vi "textParsePowerBoard.vi"(8 "error in (no error)":errorcluster, 10 "file name":string, 11 "base path":path=path "C:/specsheetsController/Sheets/PowerBoard") -> (0 "error out":errorcluster, 2 "all rows":string[][](array[string]), 3 "appended path":path)   [LabVIEW 2018]
uses:
  <vilib>/Utility/file.llb/Read Delimited Spreadsheet (string).vi
  MotorController/#include/Global textParse.vi
panel:
  out "protocolGrade":string
  out "protocolDistance":string
  out "protocolResistance":string
  out "Sense Voltage Tol. Max":string
  out "Sense Voltage Tol. Min":string
  out "Sense Voltage":string
  out "Allowable Power Interuption":string
  out "Voltage Micro Tol. Max":string
  out "Voltage Micro Tol. Min":string
  out "Voltage Micro":string
  out "Rated Output Current Tol. Max":string
  out "Rated Output Current Tol. Min":string
  out "Rated Output Current":string
  out "Ripple/Noise Tol. Max":string
  out "Ripple/Noise Tol. Min":string
  out "Ripple/Noise":string
  out "Voltage Output Tol. Max":string
  out "Voltage  Output Tol. Min":string
  out "Voltage Output":string
  out "Max Input Current":string
  out "Input Current":string
  out "Input Voltage Tol. Max":string
  out "Input Voltage Tol. Min":string
  out "Input Voltage":string
  out "Firmware":string
  out "Part Number":string
  out "Part Name":string
  # "Global variables"
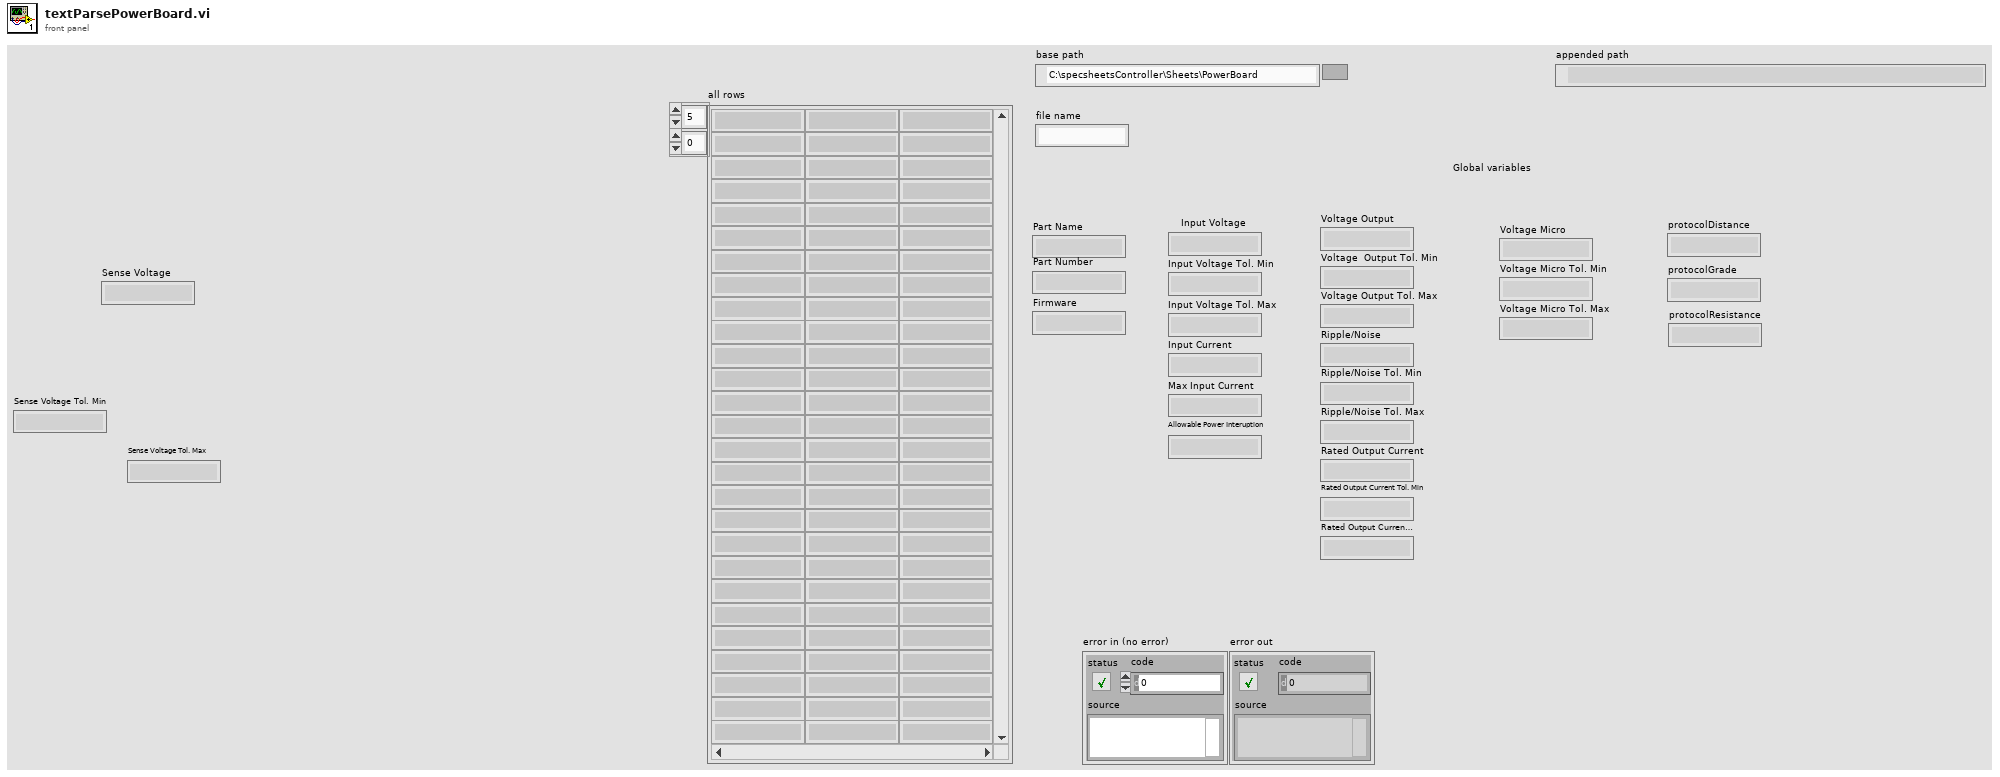
[diagram p1: front panel]
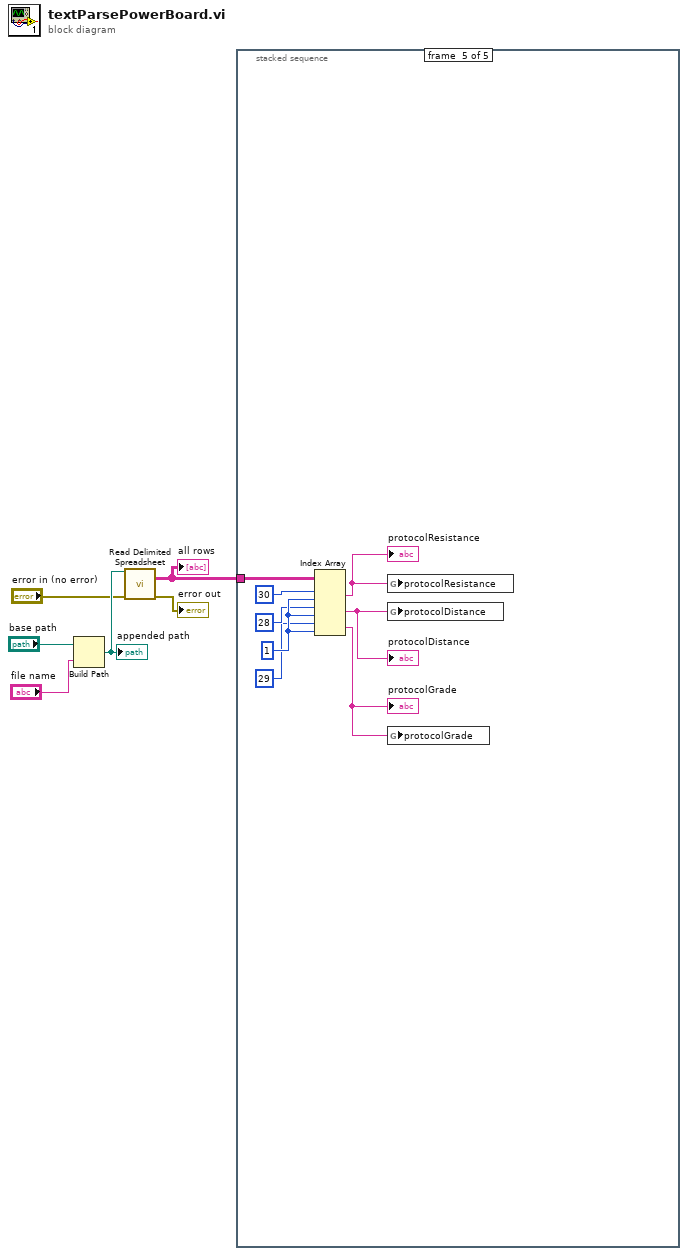
[diagram p0: block diagram]
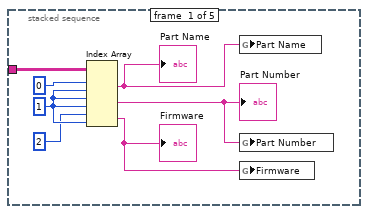
[diagram p2: hidden frame]
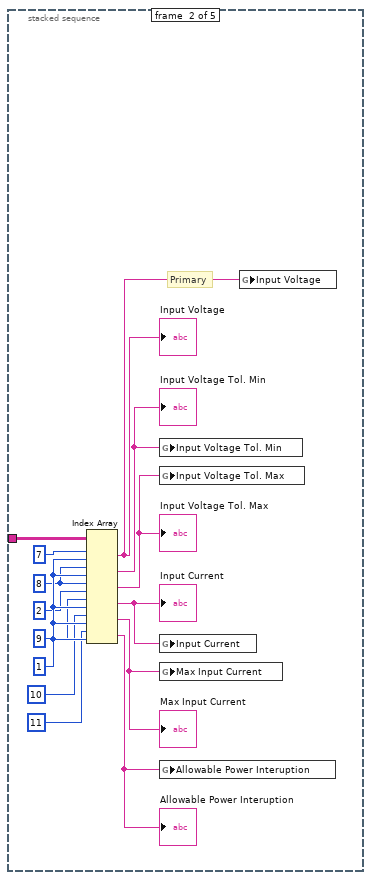
[diagram p3: hidden frame]
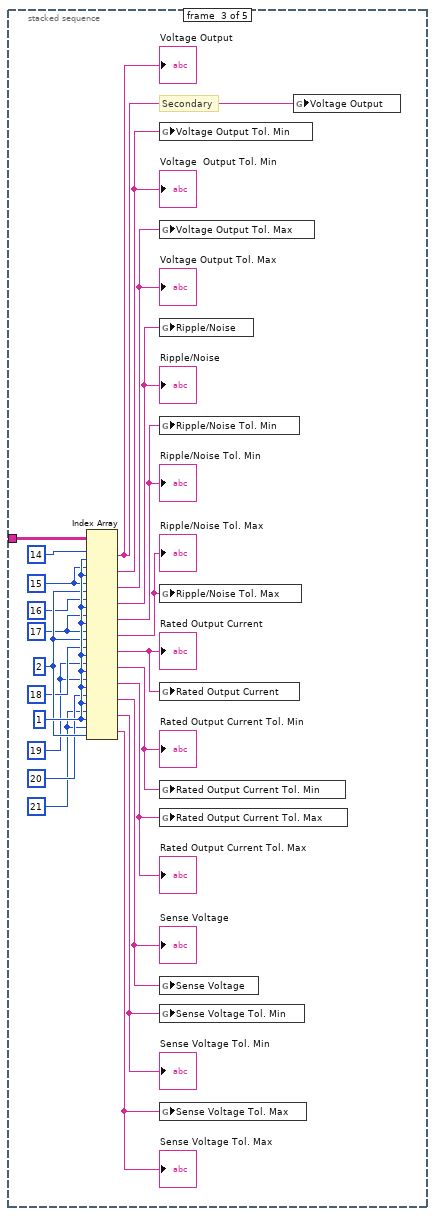
[diagram p4: hidden frame]
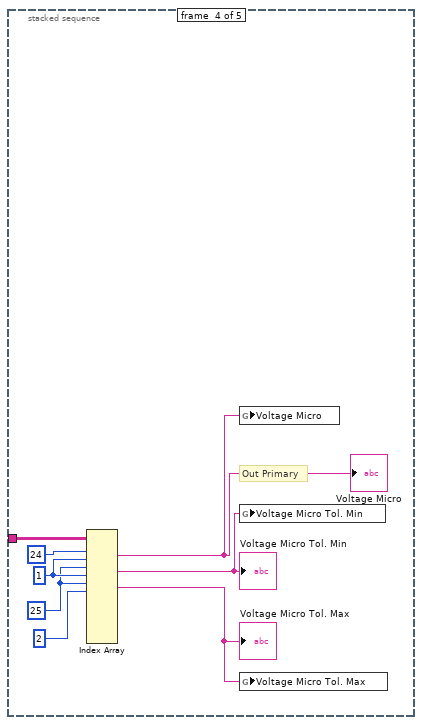
[diagram p5: hidden frame]
diagram:
  n1 = Build Path(base path="base path", name or relative path="file name") -> (appended path=w4:path)
  "appended path" <- w4
  n2 = call-poly <vilib>:"Read Delimited Spreadsheet.vi"("file path (dialog if empty)"=w4, "error in (no error)"="error in (no error)") -> ("all rows"=w1:string[][], "error out"=→"error out":errorcluster)  [unwired: 8 in, 4 out]
  "all rows" <- w1
  n3 = stacked-sequence {
    tunnel: w1 -> [w7 w14 w28 w51 w59]
    frame #0 {
      w9 = 1
      n4 = Index Array(array=w7, index (row) #1=0 ("index (row)"), index (col) #1=w9, index (row) #2=w9, index (col) #2=w9, index (row) #3=2 ("index (row)"), index (col) #3=w9) -> (element #1=w11:string, element #2=w13:string, element #3=w12:string)
      "Part Name" <- w11
      "Part Number" <- w13
      "Firmware" <- w12
      n5 = global write "Global textParse.vi" "Part Name"(w11) -> ()
      n6 = global write "Global textParse.vi" "Part Number"(w13) -> ()
      n7 = global write "Global textParse.vi" "Firmware"(w12) -> ()
    }
    frame #1 {
      w19 = 8
      w20 = 1
      # "Primary"
      n8 = Index Array(array=w14, index (row) #1=7, index (col) #1=w20, index (row) #2=w19, index (col) #2=w20, index (row) #3=w19, index (col) #3=2, index (row) #4=9, index (col) #4=w20, index (row) #5=10, index (col) #5=w20, index (row) #6=11, index (col) #6=w20) -> (element #1=w22:string, element #2=w23:string, element #3=w24:string, element #4=w25:string, element #5=w26:string, element #6=w27:string)
      "Input Voltage" <- w22
      "Input Voltage Tol. Min" <- w23
      "Input Voltage Tol. Max" <- w24
      "Input Current" <- w25
      "Max Input Current" <- w26
      "Allowable Power Interuption" <- w27
      n9 = global write "Global textParse.vi" "Input Voltage Tol. Min"(w23) -> ()
      n10 = global write "Global textParse.vi" "Input Voltage Tol. Max"(w24) -> ()
      n11 = global write "Global textParse.vi" "Input Current"(w25) -> ()
      n12 = global write "Global textParse.vi" "Max Input Current"(w26) -> ()
      n13 = global write "Global textParse.vi" "Allowable Power Interuption"(w27) -> ()
      n14 = global write "Global textParse.vi" "Input Voltage"(w22) -> ()
    }
    frame #2 {
      w29 = 21 ("index (row)")
      w31 = 19 ("index (row)")
      w37 = 1
      w35 = 2
      w33 = 17 ("index (row) 15")
      w36 = 15 ("index (row) 13")
      # "Secondary"
      n15 = Index Array(array=w28, index (row) #1=14 ("index (row) 12"), index (col) #1=w37, index (row) #2=w36, index (col) #2=w37, index (row) #3=w36, index (col) #3=w35, index (row) #4=16 ("index (row) 14"), index (col) #4=w37, index (row) #5=w33, index (col) #5=w37, index (row) #6=w33, index (col) #6=w35, index (row) #7=18 ("index (row) 19"), index (col) #7=w37, index (row) #8=w31, index (col) #8=w37, index (row) #9=w31, index (col) #9=w37, index (row) #10=20 ("index (row)"), index (col) #10=w37, index (row) #11=w29, index (col) #11=w37, index (row) #12=w29, index (col) #12=w35) -> (element #1=w42:string, element #2=w43:string, element #3=w44:string, element #4=w45:string, element #5=w46:string, element #6=w47:string, element #7=w48:string, element #8=w49:string, element #9=w50:string, element #10=w41:string, element #11=w40:string, element #12=w39:string)
      "Voltage Output" <- w42
      "Voltage  Output Tol. Min" <- w43
      "Voltage Output Tol. Max" <- w44
      "Ripple/Noise" <- w45
      "Ripple/Noise Tol. Min" <- w46
      "Ripple/Noise Tol. Max" <- w47
      "Rated Output Current" <- w48
      "Rated Output Current Tol. Min" <- w49
      "Rated Output Current Tol. Max" <- w50
      "Sense Voltage" <- w41
      "Sense Voltage Tol. Min" <- w40
      "Sense Voltage Tol. Max" <- w39
      n16 = global write "Global textParse.vi" "Voltage Output Tol. Min"(w43) -> ()
      n17 = global write "Global textParse.vi" "Voltage Output Tol. Max"(w44) -> ()
      n18 = global write "Global textParse.vi" "Ripple/Noise"(w45) -> ()
      n19 = global write "Global textParse.vi" "Ripple/Noise Tol. Min"(w46) -> ()
      n20 = global write "Global textParse.vi" "Ripple/Noise Tol. Max"(w47) -> ()
      n21 = global write "Global textParse.vi" "Rated Output Current"(w48) -> ()
      n22 = global write "Global textParse.vi" "Rated Output Current Tol. Min"(w49) -> ()
      n23 = global write "Global textParse.vi" "Rated Output Current Tol. Max"(w50) -> ()
      n24 = global write "Global textParse.vi" "Sense Voltage"(w41) -> ()
      n25 = global write "Global textParse.vi" "Sense Voltage Tol. Min"(w40) -> ()
      n26 = global write "Global textParse.vi" "Sense Voltage Tol. Max"(w39) -> ()
      n27 = global write "Global textParse.vi" "Voltage Output"(w42) -> ()
    }
    frame #3 {
      w54 = 1
      w53 = 25 ("index (row) 25")
      # "Out Primary"
      n28 = Index Array "Index Array"(array=w51, index (row) #1=24 ("index (row) 24"), index (col) #1=w54, index (row) #2=w53, index (col) #2=w54, index (row) #3=w53, index (col) #3=2) -> (element #1=w56:string, element #2=w57:string, element #3=w58:string)  [unwired: 6 in, 3 out]
      "Voltage Micro" <- w56
      "Voltage Micro Tol. Min" <- w57
      "Voltage Micro Tol. Max" <- w58
      n29 = global write "Global textParse.vi" "Voltage Micro"(w56) -> ()
      n30 = global write "Global textParse.vi" "Voltage Micro Tol. Min"(w57) -> ()
      n31 = global write "Global textParse.vi" "Voltage Micro Tol. Max"(w58) -> ()
    }
    frame #4 {
      w62 = 1 ("disabled index (col)")
      n32 = Index Array(array=w59, index (row) #1=30 ("index (row)"), index (col) #1=w62, index (row) #2=28 ("index (row)"), index (col) #2=w62, index (row) #3=29 ("index (row)"), index (col) #3=w62) -> (element #1=w64:string, element #2=w65:string, element #3=w66:string)
      "protocolResistance" <- w64
      "protocolDistance" <- w65
      "protocolGrade" <- w66
      n33 = global write "Global textParse.vi" "protocolResistance"(w64) -> ()
      n34 = global write "Global textParse.vi" "protocolDistance"(w65) -> ()
      n35 = global write "Global textParse.vi" "protocolGrade"(w66) -> ()
    }
  }
